vi "Pulse Eload.vi"(8 "error in":errorcluster, 11 "Electronic Load in":refnum<class "Electronic Load.lvclass">) -> (0 "error out":errorcluster, 3 "Electronic Load out":refnum<class "Electronic Load.lvclass">)   [LabVIEW 2019, in "Electronic Load.lvlib" / "Electronic Load.lvclass"]
uses:
  Library/Electronic Load.lvclass
  C:/Users/Public/Documents/Development/builds/Instruments/Instruments.lvlibp/Library/Instruments.lvclass
  builds/Instruments/Instruments.lvlibp/Accessors/Write Snapshot.vi
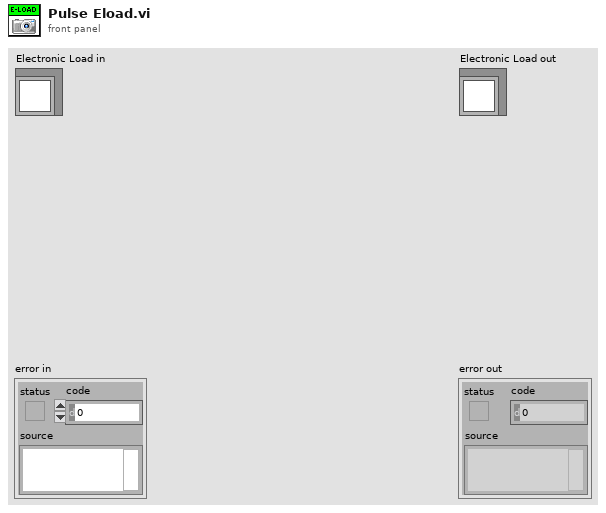
[diagram p1: front panel]
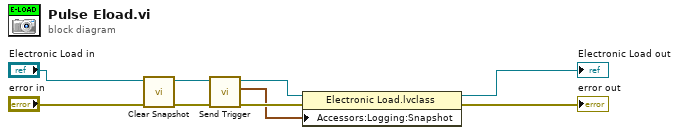
[diagram p0: block diagram]
diagram:
  n1 = call "Clear Snapshot.vi"("error in"="error in", "Electronic Load in"="Electronic Load in") -> ("error out"=w7:errorcluster, "Electronic Load out"=w6:refnum<class "Electronic Load.lvclass">)  [unwired: 8 in]
  n2 = call-dynamic "Send Trigger.vi"("error in (no error)"=w7, "Electronic Load in"=w6) -> ("error out"=w3:errorcluster, "Pulse Data"=w1:waveform(dbl)[], "Electronic Load out"=w5:refnum<class "Electronic Load.lvclass">)  [unwired: 7 in]
  n3 = property class="Electronic Load.lvclass"(reference=w5, error in=w3, "Accessors:Logging:Snapshot"=w1) -> (reference out=→"Electronic Load out":refnum<class "Electronic Load.lvclass">, error out=→"error out":errorcluster)
